vi "AMI1700eth_meas_n2_lev.vi"(8 "error in":errorcluster, 11 "conn_id_in":refnum<k5>) -> (0 "error out":errorcluster, 2 "level":dbl, 3 "conn_id_out":refnum<k5>, 4 "status":bool)   [LabVIEW 2019]
panel:
  out "string 1":string
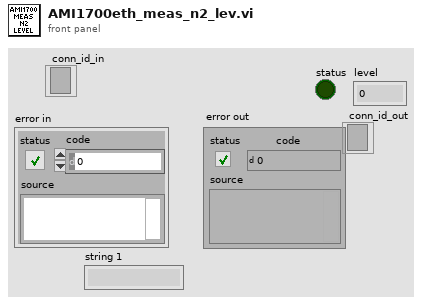
[diagram p1: front panel]
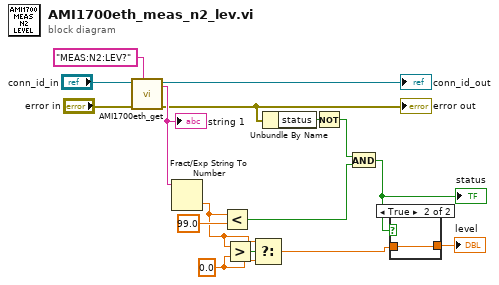
[diagram p0: block diagram]
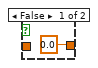
[diagram p2: hidden frame]
diagram:
  w3 = 0.0 ("f")
  n1 = call "AMI1700eth_get.vi"("command"="MEAS:N2:LEV?" ("string"), "error in"="error in", "conn_id_in"="conn_id_in") -> ("error out"=w9:errorcluster, "conn_id_out"=→"conn_id_out":refnum<k5>, "string"=w13:string)  [unwired: 5 in, 1 out]
  "error out" <- w9
  "string 1" <- w13
  n2 = Fract/Exp String To Number(string=w13) -> (number=w2:dbl)  [unwired: 3 in, 1 out]
  n3 = Less?(x=w2, y=99.0) -> (x < y?=w6:bool)
  n4 = Greater?(x=w2, y=w3) -> (0:w4:bool)
  n5 = Select(t=w2, s=w4, f=w3) -> (s? t:f=w1:dbl)
  n6 = Unbundle By Name(w9) -> ("status"=w8:bool)
  n7 = Not(x=w8) -> (.not. x?=w7:bool)
  n8 = And(x=w7, y=w6) -> (x .and. y?=w5:bool)
  "status" <- w5
  n9 = case shown="True" w5 {
    tunnel: [0.0 w18] -> w12
    tunnel: w1 -> [_ w18]
    frame False {
    }
    frame True {
    }
  }
  "level" <- w12
